vi "Definition Cluster.vi"(11 "Entity in":refnum<class "Entity.lvclass">) -> (2 "Definition":variant, 3 "Entity out":refnum<class "Entity.lvclass">)   [LabVIEW 2020, in "Conditum.lvlib" / "Columns.lvlib" / "Entity.lvclass"]
uses:
  Entity.lvclass
  Entity.lvclass/Entity.ctl
  Relation Mapping.ctl
  Conditum.lvlib
  Relation/Relation Info.ctl
  Relation/Relation.lvclass
  Type/Definition.ctl
  Type/Type.lvclass
  Relation/Relation Definition.ctl
  C:/dev/lv20CE/lv-conditum/Conditum/Columns/Relation/Relation.lvclass
  C:/dev/lv20CE/lv-conditum/Conditum/Columns/Type/Type.lvclass
  C:/dev/lv20CE/lv-conditum/Conditum/Columns/Entity/Entity.lvclass
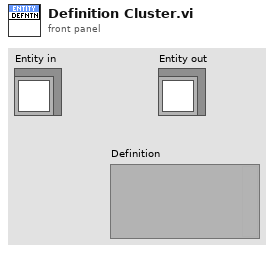
[diagram p1: front panel]
types:
  T1 = typedef "Conditum.lvlib/Columns.lvlib/Relation.lvclass/Relation Definition.ctl" = cluster{"Type":T2, "Relation":T3}
  T2 = typedef "Conditum.lvlib/Columns.lvlib/Type.lvclass/Definition.ctl" = cluster{"Name":string, "Nullable":bool, "Default NULL":bool}
  T3 = typedef "Conditum.lvlib/Relation Info.ctl" = cluster{"Mapping":T4, "Related To":string, "Reversed By":string}
  T4 = typedef "Conditum.lvlib/Relation Mapping.ctl" = enum16{"OneToMany", "ManyToOne", "ManyToMany", "OneToOne"}
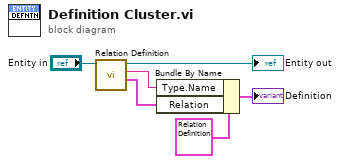
[diagram p0: block diagram]
diagram:
  n1 = call "Relation Definition.vi"("Relation in"="Entity in") -> ("Relation Definition"=w4:T3, "Table Name"=w5:string, "Relation out"=→"Entity out":refnum<class "Entity.lvclass">)  [unwired: 8 in]
  n2 = Bundle By Name(cluster=T1 {"Type"={"Name"="", "Nullable"=FALSE, "Default NULL"=FALSE}, "Relation"={"Mapping"=enum."OneToMany", "Related To"="", "Reversed By"=""}} ("Relation Definition"), "Type.Name"=w5, "Relation"=w4) -> (→"Definition":T1)
